vi "rtin_controlRealTimeInStepsPerPulse.vi"(7 "Set":bool, 8 "error in":errorcluster, 9 "Steps":i32, 10 "axis in":u8, 11 "connection ID":refnum<k5>) -> (0 "error out":errorcluster, 1 "Steps out":i32, 2 "axis out":i32, 3 "connection ID":refnum<k5>)   [LabVIEW 2016]
doc: "Sets or retrieves the change in step per pulse of the realtime input when trigger and stepper mode is used.\n Only used in open loop operation"
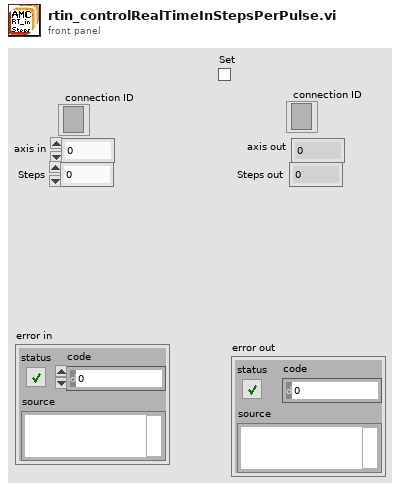
[diagram p1: front panel]
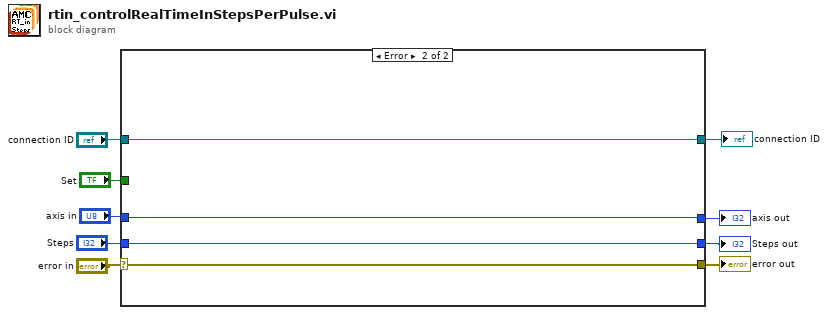
[diagram p0: block diagram]
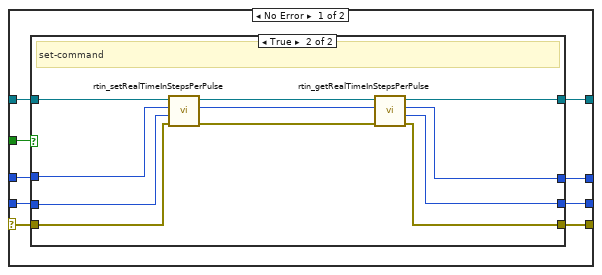
[diagram p2: hidden frame]
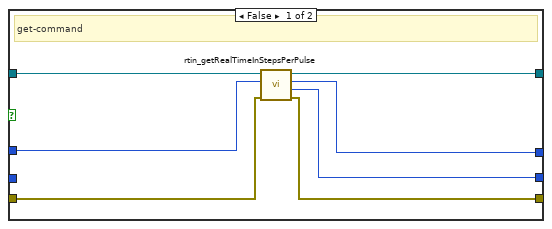
[diagram p3: hidden frame]
diagram:
  n1 = case shown="Error" "error in" {
    selector: "error in" -> [w14 w40]
    tunnel: "axis in" -> [w18 w38]
    tunnel: [w11 w40] -> w8
    tunnel: "Steps" -> [w16 w39]
    tunnel: [w13 w39] -> w3
    tunnel: "Set" -> [w15 _]
    tunnel: [w12 w37] -> w6
    tunnel: "connection ID" -> [w17 w37]
    tunnel: [w10 w38] -> w1
    frame No Error {
      n2 = case shown="True" w15 {
        tunnel: w17 -> [w25 w33]
        tunnel: w18 -> [w21 w29]
        tunnel: w16 -> [_ w28]
        tunnel: w14 -> [w22 w27]
        tunnel: [w19 w26] -> w13
        tunnel: [w24 w32] -> w12
        tunnel: [w23 w31] -> w11
        tunnel: [w20 w30] -> w10
        frame False {
          # "get-command"
          n3 = call "rtin_getRealTimeInStepsPerPulse.vi"("error in"=w22, "axis"=w21, "connection ID"=w25) -> ("error out"=w23:errorcluster, "steps"=w19:i32, "axis_out"=w20:i32, "connection ID"=w24:refnum<k5>)  [unwired: 5 in]
        }
        frame True {
          # "set-command"
          n4 = call "rtin_setRealTimeInStepsPerPulse.vi"("error in"=w27, "steps"=w28, "axis"=w29, "connection ID"=w33) -> ("error out"=w34:errorcluster, "axis_out"=w36:i32, "connection ID"=w35:refnum<k5>)  [unwired: 5 in]
          n5 = call "rtin_getRealTimeInStepsPerPulse.vi"("error in"=w34, "axis"=w36, "connection ID"=w35) -> ("error out"=w31:errorcluster, "steps"=w26:i32, "axis_out"=w30:i32, "connection ID"=w32:refnum<k5>)  [unwired: 5 in]
        }
      }
    }
    frame Error {
    }
  }
  "error out" <- w8
  "axis out" <- w1
  "Steps out" <- w3
  "connection ID" <- w6
